vi "Get Robot Pose Coordinates.vi"(0 "Intersection Points":cluster{cluster{dbl, dbl}[]}[](array[cluster]), 1 "Circle Points":T1(array[cluster]), 2 "April Tag Info":dbl[][](array[numeric]), 3 "IMU value":dbl) -> (10 "Robot Pose":cluster{dbl, dbl})   [LabVIEW 2025]
panel:
  out "Array":dbl[][](array[numeric])
  in  "Distance Deadband":dbl=0.0001 format="%#_13g"
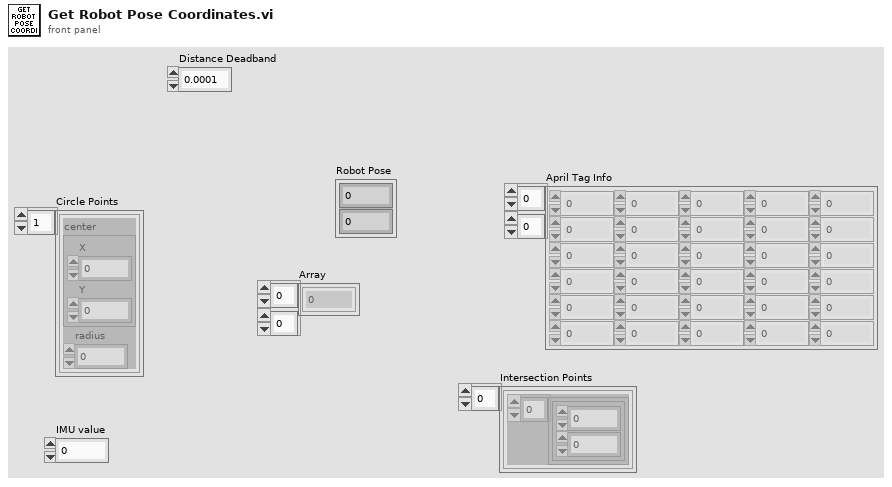
[diagram p1: front panel]
types:
  T1 = cluster{"center":cluster{"X":sgl, "Y":sgl}, "radius":sgl}[]
  T2 = cluster{"center":cluster{"X":sgl, "Y":sgl}, "radius":sgl}
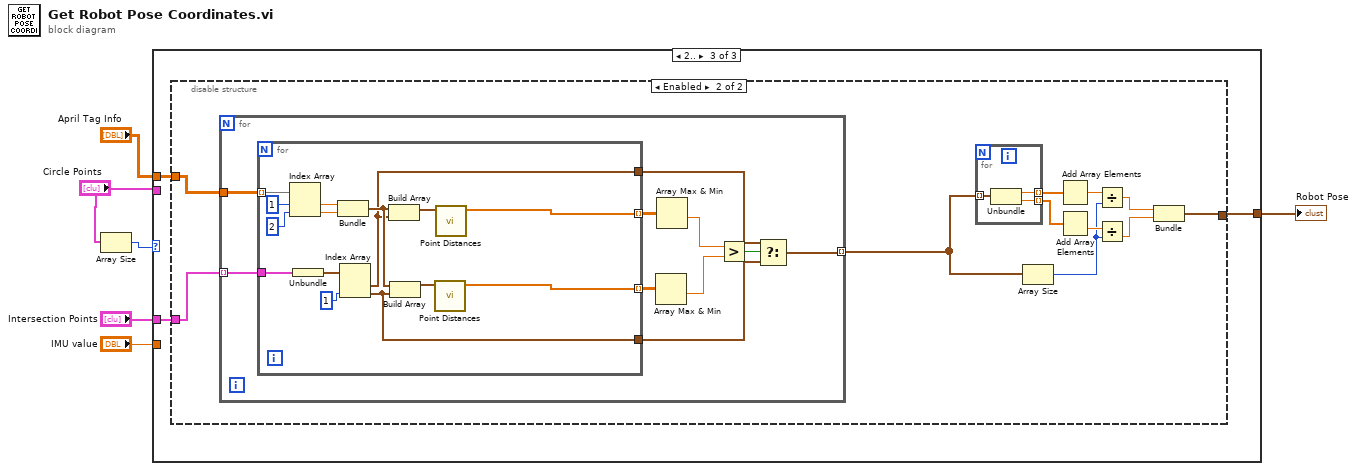
[diagram p0: block diagram]
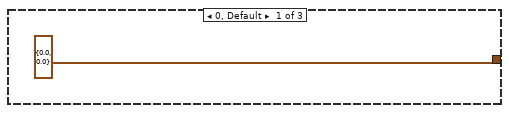
[diagram p2: hidden frame]
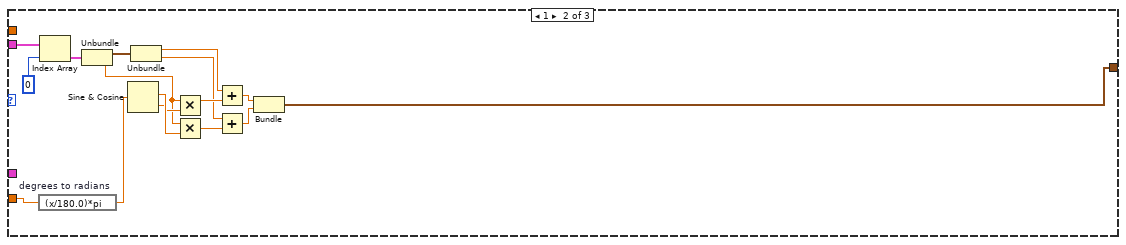
[diagram p3: hidden frame]
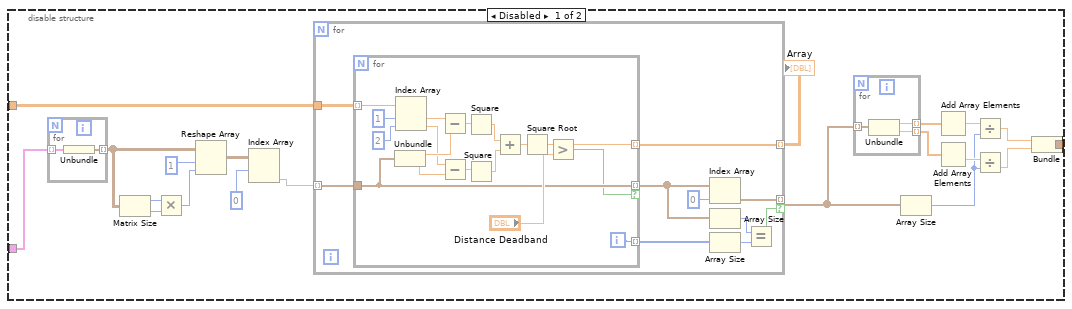
[diagram p4: hidden frame]
diagram:
  n1 = Array Size(array="Circle Points") -> (size(s)=w5:i32)
  n2 = case shown="2.." w5 {
    tunnel: "IMU value" -> [_ w23 _]
    tunnel: "Circle Points" -> [_ w22 _]
    tunnel: "Intersection Points" -> [_ _ w26]
    tunnel: [cluster{dbl, dbl} {0.0, 0.0} w10 w25] -> w2
    tunnel: "April Tag Info" -> [_ _ w24]
    frame 0, Default {
    }
    frame 1 {
      n3 = expression code="(x/180.0)*pi" "degrees to radians"(w23) -> (w18:dbl)
      n4 = Index Array(array=w22, index=0) -> (element=w20:T2)
      n5 = Unbundle(w20) -> ("center"=w19:cluster{"X":sgl, "Y":sgl}, "radius"=w13:sgl)
      n6 = Sine & Cosine(0:w18) -> (1:w17:dbl, 2:w16:dbl)
      n7 = Unbundle(w19) -> ("X"=w12:sgl, "Y"=w11:sgl)
      n8 = Multiply(x=w13, y=w16) -> (x*y=w14:dbl)
      n9 = Multiply(x=w13, y=w17) -> (x*y=w15:dbl)
      n10 = Add(x=w12, y=w14) -> (x+y=w9:dbl)
      n11 = Add(x=w11, y=w15) -> (x+y=w8:dbl)
      n12 = Bundle(w9, w8) -> (w10:cluster{dbl, dbl})  [unwired: 1 in]
    }
    frame 2.. {
      n13 = disable-structure shown="Enabled" {
        disable-tunnel: w26 -> [w46 w89]
        disable-tunnel: [w31 w79] -> w25
        disable-tunnel: w24 -> [w29 w88]
        frame Disabled {
          n14 = for {
            tunnel: w46 -> [w78] mode=indexing
            tunnel: [w77] -> w45 mode=indexing
            n15 = Unbundle(w78) -> (w77:cluster{dbl, dbl}[])
          }
          n16 = Matrix Size(0:w45) -> (1:w44:i32, 2:w43:i32)
          n17 = Multiply(x=w44, y=w43) -> (x*y=w40:i32)
          n18 = Reshape Array(w45, 1 ("dimension size"), w40) -> (w41:cluster{dbl, dbl}[][])
          n19 = Index Array(array=w41, index (row)=0 ("index")) -> (element=w30:cluster{dbl, dbl}[])  [unwired: 1 in]
          n20 = for {
            tunnel: w30 -> [w55] mode=indexing
            tunnel: w29 -> [w56]
            tunnel: [w53] -> w28 mode=indexing if=w50
            tunnel: [w47] -> w27 mode=indexing
            n21 = for {
              tunnel: w56 -> [w73] mode=indexing
              tunnel: w55 -> [w60]
              tunnel: [w60] -> w49 mode=indexing if=w59
              tunnel: [w58] -> w48 mode=indexing
              tunnel: [w57] -> w47 mode=indexing
              i -> [w58]
              n22 = Unbundle(w60) -> (w69:dbl, w67:dbl)
              n23 = Index Array(array=w73, index #1=1 ("index"), index #2=2 ("index")) -> (element #1=w70:dbl, element #2=w68:dbl)
              n24 = Subtract(x=w70, y=w69) -> (x-y=w66:dbl)
              n25 = Subtract(x=w68, y=w67) -> (x-y=w65:dbl)
              n26 = Square(x=w66) -> (x^2=w64:dbl)
              n27 = Square(x=w65) -> (x^2=w63:dbl)
              n28 = Add(x=w64, y=w63) -> (x+y=w62:dbl)
              n29 = Square Root(x=w62) -> (sqrt(x)=w57:dbl)
              n30 = Greater?(x=w57, y="Distance Deadband") -> (0:w59:bool)
            }
            n31 = Index Array(array=w49, index=0) -> (element=w53:cluster{dbl, dbl})
            n32 = Array Size(array=w49) -> (size(s)=w52:i32)
            n33 = Array Size(array=w48) -> (size(s)=w51:i32)
            n34 = Equal?(x=w52, y=w51) -> (x = y?=w50:bool)
          }
          "Array" <- w27
          n35 = for {
            tunnel: w28 -> [w76] mode=indexing
            tunnel: [w75] -> w38 mode=indexing
            tunnel: [w74] -> w37 mode=indexing
            n36 = Unbundle(w76) -> (w75:dbl, w74:dbl)
          }
          n37 = Array Size(array=w28) -> (size(s)=w34:i32)
          n38 = Add Array Elements(numeric array=w38) -> (sum=w36:dbl)
          n39 = Add Array Elements(numeric array=w37) -> (sum=w35:dbl)
          n40 = Divide(x=w36, y=w34) -> (x/y=w33:dbl)
          n41 = Divide(x=w35, y=w34) -> (x/y=w32:dbl)
          n42 = Bundle(w33, w32) -> (w31:cluster{dbl, dbl})  [unwired: 1 in]
        }
        frame Enabled {
          n43 = for {
            tunnel: w89 -> [w101] mode=indexing
            tunnel: w88 -> [w102]
            tunnel: [w93] -> w80 mode=indexing
            n44 = for {
              tunnel: w102 -> [w117] mode=indexing
              tunnel: w101 -> [w114]
              tunnel: [w106] -> w100 mode=indexing
              tunnel: [w105] -> w99 mode=indexing
              tunnel: [w104] -> w97
              tunnel: [w103] -> w98
              n45 = Index Array(array=w117, index #1=1 ("index"), index #2=2 ("index")) -> (element #1=w111:dbl, element #2=w110:dbl)
              n46 = Unbundle(w114) -> (w113:cluster{dbl, dbl}[])
              n47 = Bundle(w111, w110) -> (w109:cluster{dbl, dbl})  [unwired: 1 in]
              n48 = Index Array(array=w113, index #2=1 ("index")) -> (element #1=w103:cluster{dbl, dbl}, element #2=w104:cluster{dbl, dbl})  [unwired: 1 in]
              n49 = Build Array(w109, w103) -> (w108:cluster{dbl, dbl}[])
              n50 = Build Array(w109, w104) -> (w107:cluster{dbl, dbl}[])
              n51 = call "Point Distances.vi"("Points"=w107) -> ("Distances"=w105:sgl[])  [unwired: 10 in]
              n52 = call "Point Distances.vi"("Points"=w108) -> ("Distances"=w106:sgl[])  [unwired: 10 in]
            }
            n53 = Array Max & Min(array=w99) -> (min value=w94:sgl)  [unwired: 3 out]
            n54 = Array Max & Min(array=w100) -> (min value=w95:sgl)  [unwired: 3 out]
            n55 = Greater?(x=w95, y=w94) -> (0:w96:bool)
            n56 = Select(t=w98, s=w96, f=w97) -> (s? t:f=w93:cluster{dbl, dbl})
          }
          n57 = for {
            tunnel: w80 -> [w92] mode=indexing
            tunnel: [w91] -> w87 mode=indexing
            tunnel: [w90] -> w86 mode=indexing
            n58 = Unbundle(w92) -> (w91:dbl, w90:dbl)
          }
          n59 = Array Size(array=w80) -> (size(s)=w83:i32)
          n60 = Add Array Elements(numeric array=w87) -> (sum=w85:dbl)
          n61 = Add Array Elements(numeric array=w86) -> (sum=w84:dbl)
          n62 = Divide(x=w85, y=w83) -> (x/y=w82:dbl)
          n63 = Divide(x=w84, y=w83) -> (x/y=w81:dbl)
          n64 = Bundle(w82, w81) -> (w79:cluster{dbl, dbl})  [unwired: 1 in]
        }
      }
    }
  }
  "Robot Pose" <- w2
